vi "Read Pulse Amplitude Power.vi"(8 "error in (no error)":errorcluster, 10 "Pulse Block (1: 1)":i32(ring)=1 items=["1"=1, "2"=2, "3"=3, "4"=4, "5"=5, "6"=6, "7"=7, "8"=8, "9"=9, "10"=10, "11"=11, "12"=12, "13"=13, "14"=14, "15"=15, "16"=16, "17"=17, "18"=18, "19"=19, "20"=20], 11 "VISA resource name":refnum<visa-resource-name>) -> (0 "error out":errorcluster, 1 "Trailing Edge Amplitude":dbl, 2 "Rising Pulse Amplitude":dbl, 3 "VISA resource name out":refnum<visa-resource-name>, 5 "Pulse Tilt":dbl)   [LabVIEW 2018, in "Agilent U2000 Series.lvlib"]
doc: "Reads pulse amplitude power.\n\nNote: \nThis VI is only applicable for U2042XA/U2044XA/U2049XA."
uses:
  Agilent U2000 Series.lvlib
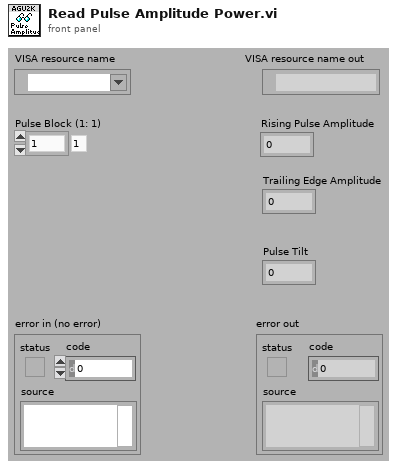
[diagram p1: front panel]
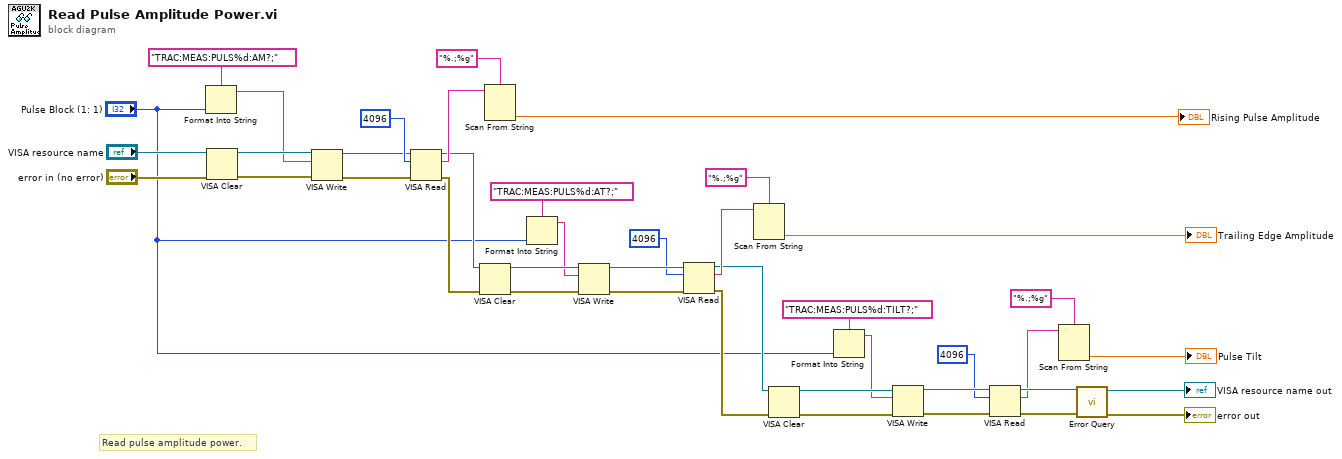
[diagram p0: block diagram]
diagram:
  # "Read pulse amplitude power."
  n1 = Format Into String(format string="TRAC:MEAS:PULS%d:AM?;", "Pulse Block (1: 1)") -> (resulting string=w34:string)  [unwired: 2 in, 1 out]
  n2 = VISA Clear(VISA resource name="VISA resource name", error in (no error)="error in (no error)") -> (VISA resource name out=w36:refnum<visa-resource-name>, error out=w35:errorcluster)
  n3 = VISA Write(VISA resource name=w36, write buffer=w34, error in (no error)=w35) -> (VISA resource name out=w33:refnum<visa-resource-name>, error out=w32:errorcluster)  [unwired: 1 out]
  n4 = VISA Read(VISA resource name=w33, byte count=u32 4096, error in (no error)=w32) -> (VISA resource name out=w28:refnum<visa-resource-name>, read buffer=w31:string, error out=w27:errorcluster)  [unwired: 1 out]
  n5 = VISA Clear(VISA resource name=w28, error in (no error)=w27) -> (VISA resource name out=w25:refnum<visa-resource-name>, error out=w24:errorcluster)
  n6 = Scan From String(format string="%.;%g", input string=w31) -> (output 1=→"Rising Pulse Amplitude":dbl)  [unwired: 3 in, 3 out]
  n7 = Format Into String(format string="TRAC:MEAS:PULS%d:AT?;", "Pulse Block (1: 1)") -> (resulting string=w21:string)  [unwired: 2 in, 1 out]
  n8 = VISA Write(VISA resource name=w25, write buffer=w21, error in (no error)=w24) -> (VISA resource name out=w23:refnum<visa-resource-name>, error out=w22:errorcluster)  [unwired: 1 out]
  n9 = VISA Read(VISA resource name=w23, byte count=u32 4096, error in (no error)=w22) -> (VISA resource name out=w16:refnum<visa-resource-name>, read buffer=w18:string, error out=w15:errorcluster)  [unwired: 1 out]
  n10 = Scan From String(format string="%.;%g", input string=w18) -> (output 1=→"Trailing Edge Amplitude":dbl)  [unwired: 3 in, 3 out]
  n11 = VISA Clear(VISA resource name=w16, error in (no error)=w15) -> (VISA resource name out=w13:refnum<visa-resource-name>, error out=w12:errorcluster)
  n12 = Format Into String(format string="TRAC:MEAS:PULS%d:TILT?;", "Pulse Block (1: 1)") -> (resulting string=w10:string)  [unwired: 2 in, 1 out]
  n13 = VISA Write(VISA resource name=w13, write buffer=w10, error in (no error)=w12) -> (VISA resource name out=w9:refnum<visa-resource-name>, error out=w8:errorcluster)  [unwired: 1 out]
  n14 = VISA Read(VISA resource name=w9, byte count=u32 4096, error in (no error)=w8) -> (VISA resource name out=w5:refnum<visa-resource-name>, read buffer=w2:string, error out=w4:errorcluster)  [unwired: 1 out]
  n15 = Scan From String(format string="%.;%g", input string=w2) -> (output 1=→"Pulse Tilt":dbl)  [unwired: 3 in, 3 out]
  n16 = call "Error Query.vi"("error in (no error)"=w4, "VISA resource name"=w5) -> ("error out"=→"error out":errorcluster, "VISA resource name out"=→"VISA resource name out":refnum<visa-resource-name>)  [unwired: 6 in, 2 out]
